vi "Scanner-Indentify-All-Action_Api.vi"(4 "加速度 (回頭)":dbl=700.0 format="%#_13g", 6 "最高速 (回頭)":dbl=800.0 format="%#_13g", 7 "Barcode數量":i32, 8 "Error In":errorcluster, 9 "加速度":dbl=700.0 format="%#_13g", 11 "最高速":dbl=800.0 format="%#_13g") -> (0 "error out":errorcluster, 1 "辨識機率":dbl[](array[slide]) scale=0.0..5.0, 2 "辨識機率":T1, 3 "輸出顏色-位置":T2(array[cluster]), 5 "總辨識結果":string[](array[string]))   [LabVIEW 2019]
uses:
  <vilib>/myRIO/Instrument Drivers/Onboard IO/DIO/typedefs/DIO Reference.ctl
  <vilib>/myRIO/Common/Instrument Driver Framework/Utilities/typedefs/myRIO Generic Hardware Reference.ctl
  <vilib>/myRIO/Common/Instrument Driver Framework/Utilities/typedefs/Hardware Version Enum.ctl
  <vilib>/myRIO/Common/Instrument Driver Framework/Utilities/typedefs/myRIO v1.0 Reference.ctl
  <vilib>/myRIO/Common/Instrument Driver Framework/Utilities/typedefs/Generic FPGA Reference.ctl
  <vilib>/myRIO/Common/Instrument Driver Framework/myRIO v1.0/DIO/typedefs/DIO Channels List.ctl
  <vilib>/myRIO/Common/Instrument Driver Framework/myRIO v1.0/DIO/typedefs/DIO Channels Enum.ctl
  <vilib>/userDefined/High Color/nirio_resource_hc.ctl
  <vilib>/myRIO/Common/Instrument Driver Framework/Utilities/vis/Is FPGA Ref Available.vi
  <vilib>/myRIO/Common/Instrument Driver Framework/myRIO v1.0/DIO/vis/myRIO v1.1 Open DIO.vi
  <vilib>/myRIO/Instrument Drivers/Onboard IO/DIO/vis/Write.vi
  b00342f0-89ff-48b8-870a-2e0bf58d2d45.vi
  <vilib>/myRIO/Common/Instrument Driver Framework/Utilities/vis/Validate Channels.vi
  <vilib>/myRIO/Common/Instrument Driver Framework/myRIO v1.0/DIO/vis/myRIO v1.0 Reserve DIO.vi
  <vilib>/myRIO/Common/Instrument Driver Framework/myRIO v1.0/Resource Manager/vis/myRIO v1.0 Reserve Channel List.vi
  <vilib>/myRIO/Common/Instrument Driver Framework/myRIO v1.0/DIO/vis/myRIO v1.0 Build MUX Configuration DIO.vi
  <vilib>/myRIO/Common/Instrument Driver Framework/myRIO v1.0/Resource Manager/vis/myRIO v1.0 Reserve Channel.vi
  <vilib>/myRIO/Common/Instrument Driver Framework/myRIO v1.0/Resource Manager/vis/myRIO v1.0 Unreserve Channel.vi
  <vilib>/myRIO/Common/Instrument Driver Framework/myRIO v1.0/Resource Manager/vis/myRIO v1.0 Create Configuration List.vi
  <vilib>/myRIO/Common/Instrument Driver Framework/myRIO v1.0/Resource Manager/vis/myRIO v1.0 Build Mutex Name.vi
  <vilib>/Utility/VariantDataType/GetNumericInfo.vi
  <vilib>/Utility/error.llb/Error Cluster From Error Code.vi
  <vilib>/myRIO/Common/Instrument Driver Framework/myRIO v1.0/myRIO v1.1 Open.vi
  <vilib>/myRIO/Common/Instrument Driver Framework/Utilities/vis/IO Manager.vi
  <vilib>/myRIO/Common/Instrument Driver Framework/Utilities/vis/Configuration Manager.vi
  <vilib>/myRIO/Common/Instrument Driver Framework/myRIO v1.0/Resource Manager/vis/myRIO v1.0 Configure IO.vi
  <vilib>/myRIO/Common/Instrument Driver Framework/myRIO v1.0/myRIO v1.0 Close.vi
  <vilib>/myRIO/Common/Instrument Driver Framework/myRIO v1.0/DIO/vis/myRIO v1.0 Write DIO.vi
  <vilib>/myRIO/Express VI/Onboard Devices/LED/LED Express VI.xnode
  <vilib>/myRIO/Instrument Drivers/Onboard IO/DIO/vis/myRIO DIO Open.xnode
  <vilib>/myRIO/Instrument Drivers/Onboard IO/DIO/DIO.lvlib
panel:
  in  "Tab Control":enum32{"Page 1", "Page 2", "Page 3"}(tab)
  out "第一次辨識機率":i32[](graph)
  out "第二次辨識結果":i32[](graph)
  out "總辨識機率 2":i32[](graph)
  out "總辨識機率":i32[](array[numeric])
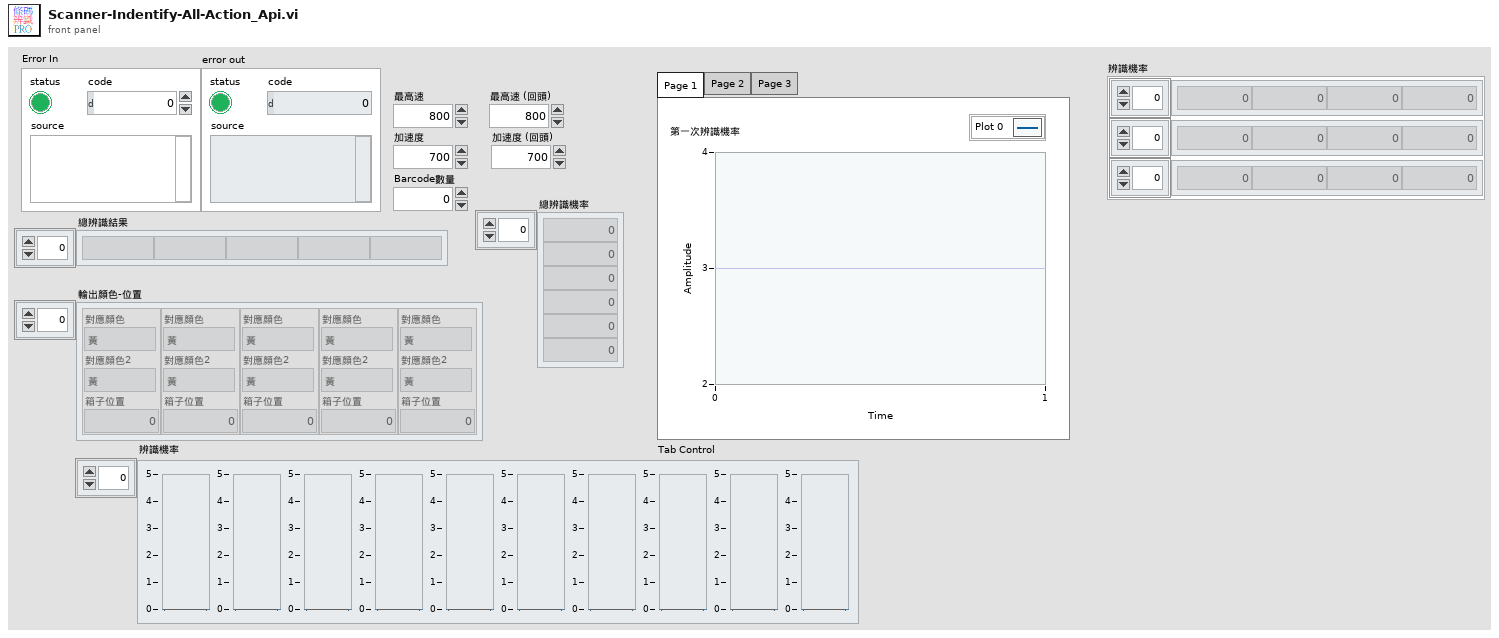
[diagram p1: front panel]
types:
  T1 = cluster{"Array":i32[], "Array":i32[], "Array":i32[]}
  T2 = cluster{"對應顏色":enum16{"黃", "紅", "綠", "藍", "黑", "無"}, "對應顏色2":enum16{"黃", "紅", "綠", "藍", "黑", "無"}, "箱子位置":i32}[]
  T3 = enum16{"前", "後", "オ", "右", "無", "0", "1", "2", "3", "4", "5", "6", "7"}
  T4 = typedef "DIO.lvlib/DIO Reference.ctl" = cluster{"myRIO Reference":T5, "DIO Channels List":T9}
  T5 = typedef "myRIO Generic Hardware Reference.ctl" = cluster{"myRIO Model":T6, "myRIO Hardware Reference":T7}
  T6 = typedef "Hardware Version Enum.ctl" = enum16{"Unknown", "myRIO-1900", "myRIO-1950", "roboRIO", "NI ELVIS RIO CM", "ELVIS III"}
  T7 = typedef "myRIO v1.0 Reference.ctl" = cluster{"Generic FPGA Reference":T8, "Allow multiple opens":bool}
  T8 = typedef "Generic FPGA Reference.ctl" = refnum<k20>
  T9 = typedef "DIO Channels List.ctl" = T10[]
  T10 = typedef "DIO Channels Enum.ctl" = enum16{"Not Connected", "C/DIO0", "C/DIO1", "C/DIO2", "C/DIO3", "C/DIO4", "C/DIO5", "C/DIO6", "C/DIO7", "A/DIO0", "A/DIO1", "A/DIO2", "A/DIO3", "A/DIO4", "A/DIO5", "A/DIO6", "A/DIO7", "A/DIO8", "A/DIO9", "A/DIO10", "A/DIO11", "A/DIO12", "A/DIO13", "A/DIO14", "A/DIO15", "A/DIO16", "A/DIO17", "A/DIO18", "A/DIO19", "B/DIO0", "B/DIO1", "B/DIO2", "B/DIO3", "B/DIO4", "B/DIO5", "B/DIO6", "B/DIO7", "B/DIO8", "B/DIO9", "B/DIO10", "B/DIO11", "B/DIO12", "B/DIO13", "B/DIO14", "B/DIO15", "B/DIO16", "B/DIO17", "B/DIO18", "B/DIO19", "LED0", "LED1", "LED2", "LED3", "Button0", "DIO/DIO0", "DIO/DIO1", "DIO/DIO2", "DIO/DIO3", "DIO/DIO4", "DIO/DIO5", "DIO/DIO6", "DIO/DIO7", "DIO/DIO8", "DIO/DIO9", "SPI/CS0", "SPI/CS1", "SPI/CS2", "SPI/CS3", "LED RADIO (Green)", "LED RADIO (Red)", "LED COMM (Green)", "LED COMM (Red)", "LED MODE (Green)", "LED MODE (Red)"}
  T11 = typedef "nirio_resource_hc.ctl" = tag
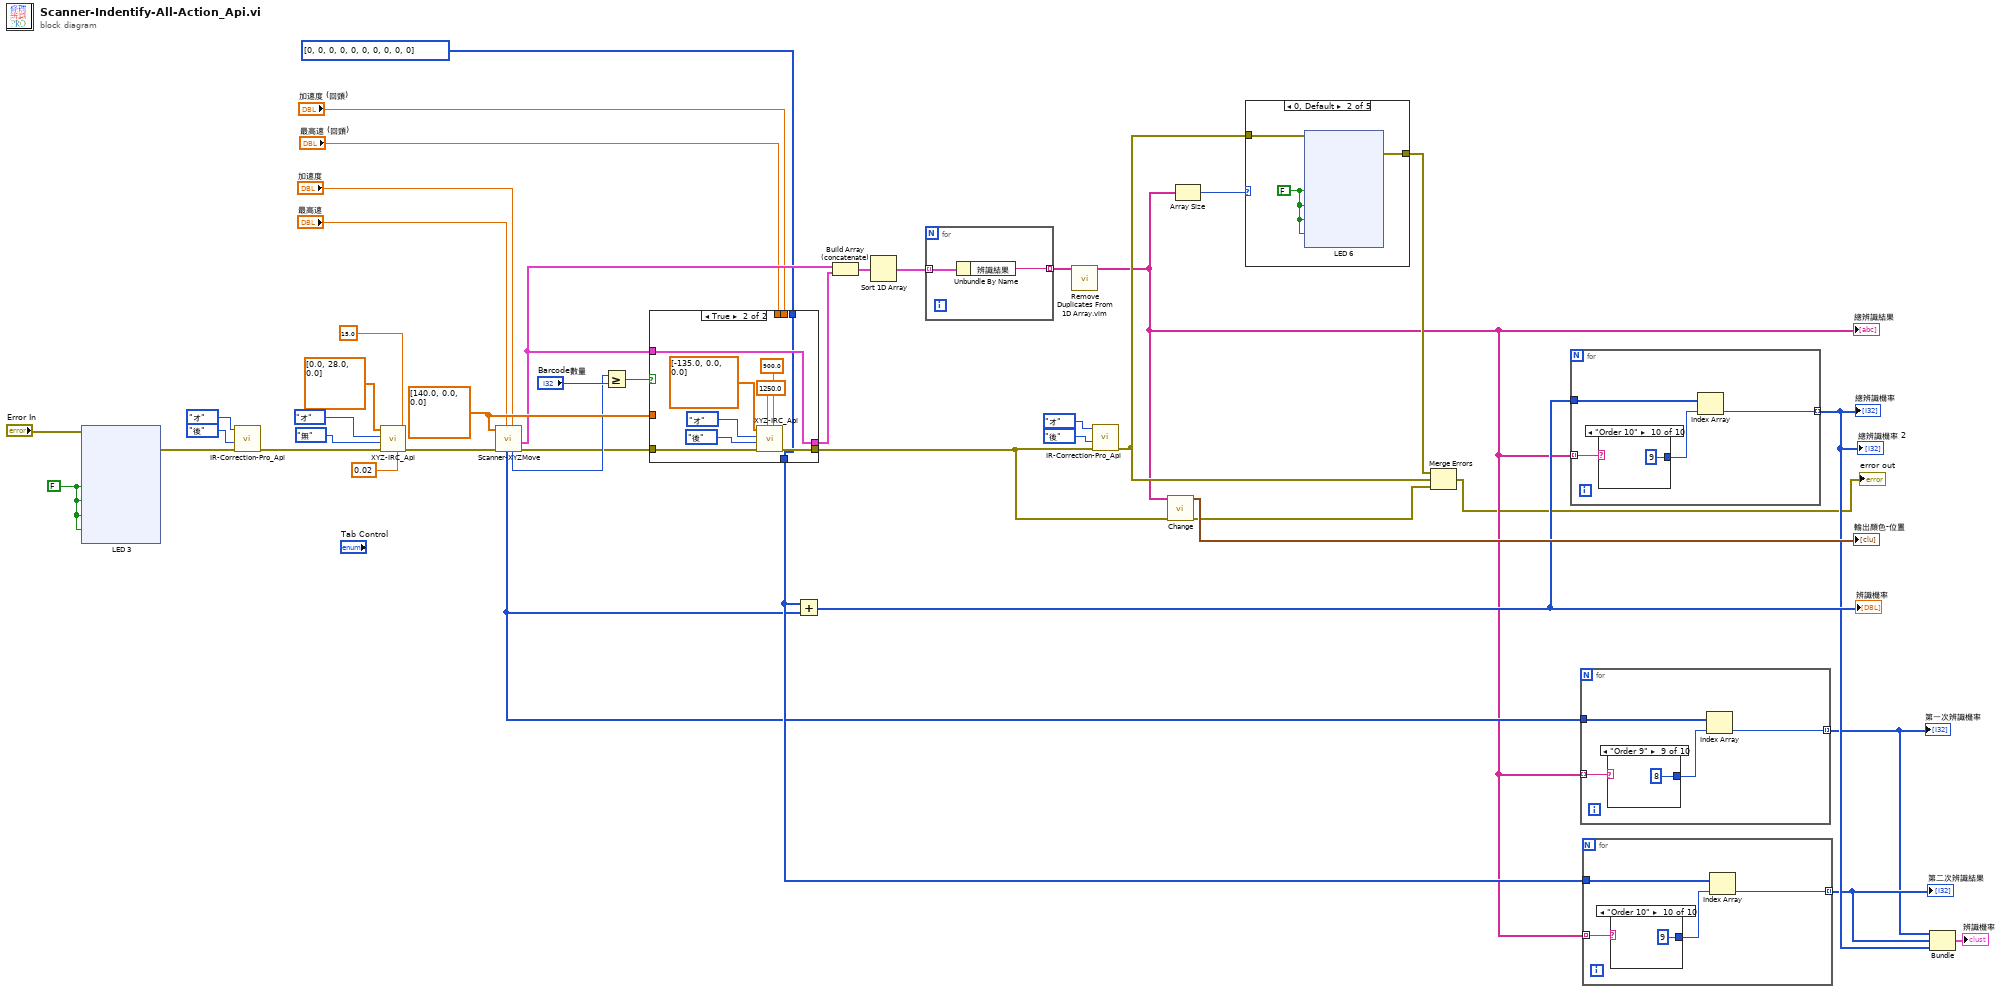
[diagram p0: block diagram]
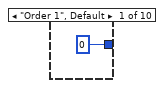
[diagram p2: hidden frame]
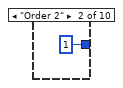
[diagram p3: hidden frame]
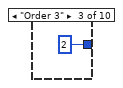
[diagram p4: hidden frame]
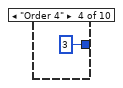
[diagram p5: hidden frame]
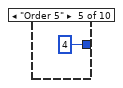
[diagram p6: hidden frame]
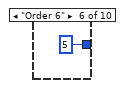
[diagram p7: hidden frame]
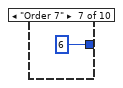
[diagram p8: hidden frame]
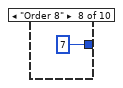
[diagram p9: hidden frame]
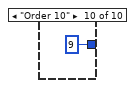
[diagram p10: hidden frame]
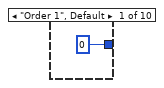
[diagram p11: hidden frame]
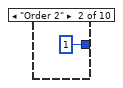
[diagram p12: hidden frame]
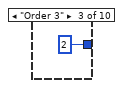
[diagram p13: hidden frame]
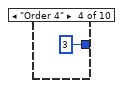
[diagram p14: hidden frame]
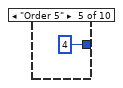
[diagram p15: hidden frame]
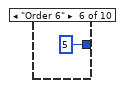
[diagram p16: hidden frame]
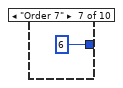
[diagram p17: hidden frame]
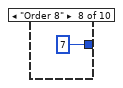
[diagram p18: hidden frame]
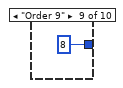
[diagram p19: hidden frame]
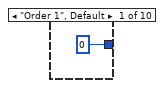
[diagram p20: hidden frame]
diagram:
  w21 = FALSE ("LED3")
  w42 = dbl[] [140.0, 0.0, 0.0] ("X-Y-Z移動")
  n1 = xnode "LED 3"("LED0"=w21, "LED1"=w21, "LED2"=w21, "LED3"=w21, "error in (no error)"="Error In") -> ("error out"=w19:errorcluster)
  n2 = call "IR-Correction-Pro_Api.vi"("Error In"=w19, "副邊校正"=T3."後", "主編校正"=enum16{"前", "後", "オ", "右", "無"}."オ") -> ("Error Out"=w32:errorcluster)  [unwired: 8 in]
  n3 = call "XYZ-IRC_Api.vi"("精準度"=15.0, "ExitRange"=0.02, "Error"=w32, "副邊校正"=T3."無", "主編校正"=enum16{"前", "後", "オ", "右", "無"}."オ", "X-Y-Z移動"=dbl[] [0.0, 28.0, 0.0]) -> ("Error Out"=w29:errorcluster)  [unwired: 5 in]
  n4 = call "Scanner-XYZMove.vi"("加速度"="加速度", "最高速"="最高速", "Error In"=w29, "X-Y-Z移動"=w42) -> ("Error Out"=w9:errorcluster, "辨識結果(包含位置)"=w18:cluster{"讀取到時的位子":dbl, "辨識結果":string}[], "辨識數量"=w15:i32, "讀取機率"=w4:i32[])  [unwired: 2 in, 2 out]
  n5 = Greater Or Equal?(x=w15, y="Barcode數量") -> (x >= y?=w16:bool)
  n6 = case shown="True" w16 {
    tunnel: w42 -> [w51 _]
    tunnel: [w50 w59] -> w40
    tunnel: [w49 w60] -> w37
    tunnel: w9 -> [w48 w61]
    tunnel: w18 -> [_ w59]
    tunnel: "加速度 (回頭)" -> [w47 _]
    tunnel: "最高速 (回頭)" -> [w46 _]
    tunnel: [w45 w53] -> w8
    tunnel: i32[] [0, 0, 0, 0, 0, 0, 0, 0, 0, 0] -> [_ w53]
    frame False {
      n7 = call "Scanner-XYZ-Back.vi"("加速度"=w47, "最高速"=w46, "Error In"=w48, "第一次位移"=w51, "X-Y-Z移動"=dbl[] [-140.0, 0.0, 0.0]) -> ("Error Out"=w49:errorcluster, "辨識結果(包含位置)"=w50:cluster{"讀取到時的位子":dbl, "辨識結果":string}[], "辨識機率"=w45:i32[])  [unwired: 2 in, 2 out]
    }
    frame True {
      n8 = call "XYZ-IRC_Api.vi"("加速度"=900.0, "最高速"=1250.0, "Error"=w61, "副邊校正"=T3."後", "主編校正"=enum16{"前", "後", "オ", "右", "無"}."オ", "X-Y-Z移動"=dbl[] [-135.0, 0.0, 0.0]) -> ("Error Out"=w60:errorcluster)  [unwired: 5 in]
    }
  }
  n9 = Add(x=w8, y=w4) -> (x+y=w10:i32[])
  "辨識機率" <- w10
  n10 = Build Array (concatenate)(w18, w40) -> (w41:cluster{"讀取到時的位子":dbl, "辨識結果":string}[])
  n11 = Sort 1D Array(array=w41) -> (sorted array=w39:cluster{"讀取到時的位子":dbl, "辨識結果":string}[])
  n12 = for {
    tunnel: w39 -> [w63] mode=indexing
    tunnel: [w62] -> w38 mode=indexing
    n13 = Unbundle By Name(w63) -> ("辨識結果"=w62:string)
  }
  n14 = call "Remove Duplicates From 1D Array.vim"("array"=w38) -> ("array with duplicates removed"=w2:string[])  [unwired: 10 in]
  "總辨識結果" <- w2
  n15 = call "IR-Correction-Pro_Api.vi"("Error In"=w37, "副邊校正"=T3."後", "主編校正"=enum16{"前", "後", "オ", "右", "無"}."オ") -> ("Error Out"=w28:errorcluster)  [unwired: 8 in]
  n16 = call "Change.vi"("Error In"=w37, "總辨識結果"=w2) -> ("Error Out"=w35:errorcluster, "輸出顏色-位置"=→"輸出顏色-位置":T2)  [unwired: 8 in]
  n17 = Array Size(array=w2) -> (size(s)=w31:i32)
  n18 = case shown="0, Default" w31 {
    tunnel: w28 -> [w66 w107 w147 w185 w225]
    tunnel: [w65 w106 w146 w184 w224] -> w30
    frame 4 {
      w64 = TRUE ("LED3")
      n19 = xnode "LED"("LED0"=w64, "LED1"=w64, "LED2"=w64, "LED3"=w64, "error in (no error)"=w66) -> ("error out"=w65:errorcluster)
    }
    frame 0, Default {
      w105 = FALSE ("LED2")
      n20 = xnode "LED 6"("LED0"=w105, "LED1"=w105, "LED2"=w105, "LED3"=w105, "error in (no error)"=w107) -> ("error out"=w106:errorcluster)
    }
    frame 1 {
      n21 = xnode "LED 5"("LED0"=TRUE ("LED2"), "error in (no error)"=w147) -> ("error out"=w146:errorcluster)
    }
    frame 2 {
      w186 = TRUE ("LED2")
      n22 = xnode "LED 4"("LED0"=w186, "LED1"=w186, "error in (no error)"=w185) -> ("error out"=w184:errorcluster)
    }
    frame 3 {
      w223 = TRUE ("LED2")
      n23 = xnode "LED 2"("LED0"=w223, "LED1"=w223, "LED2"=w223, "error in (no error)"=w225) -> ("error out"=w224:errorcluster)
    }
  }
  n24 = Merge Errors(w30, w28, w35) -> (→"error out":errorcluster)
  n25 = for {
    tunnel: w2 -> [w266] mode=indexing
    tunnel: w10 -> [w265]
    tunnel: [w263] -> w7 mode=indexing
    n26 = case shown="\"Order 10\"" w266 {
      tunnel: [0 1 2 3 4 5 6 7 8 9] -> w264
      frame "Order 1", Default {
      }
      frame "Order 2" {
      }
      frame "Order 3" {
      }
      frame "Order 4" {
      }
      frame "Order 5" {
      }
      frame "Order 6" {
      }
      frame "Order 7" {
      }
      frame "Order 8" {
      }
      frame "Order 9" {
      }
      frame "Order 10" {
      }
    }
    n27 = Index Array(array=w265, index=w264) -> (element=w263:i32)
  }
  "總辨識機率" <- w7
  "總辨識機率 2" <- w7
  n28 = for {
    tunnel: w4 -> [w280]
    tunnel: [w278] -> w3 mode=indexing
    tunnel: w2 -> [w277] mode=indexing
    n29 = case shown="\"Order 9\"" w277 {
      tunnel: [0 1 2 3 4 5 6 7 8 9] -> w279
      frame "Order 1", Default {
      }
      frame "Order 2" {
      }
      frame "Order 3" {
      }
      frame "Order 4" {
      }
      frame "Order 5" {
      }
      frame "Order 6" {
      }
      frame "Order 7" {
      }
      frame "Order 8" {
      }
      frame "Order 9" {
      }
      frame "Order 10" {
      }
    }
    n30 = Index Array(array=w280, index=w279) -> (element=w278:i32)
  }
  "第一次辨識機率" <- w3
  n31 = for {
    tunnel: w8 -> [w294]
    tunnel: [w292] -> w6 mode=indexing
    tunnel: w2 -> [w291] mode=indexing
    n32 = case shown="\"Order 10\"" w291 {
      tunnel: [0 1 2 3 4 5 6 7 8 9] -> w293
      frame "Order 1", Default {
      }
      frame "Order 2" {
      }
      frame "Order 3" {
      }
      frame "Order 4" {
      }
      frame "Order 5" {
      }
      frame "Order 6" {
      }
      frame "Order 7" {
      }
      frame "Order 8" {
      }
      frame "Order 9" {
      }
      frame "Order 10" {
      }
    }
    n33 = Index Array(array=w294, index=w293) -> (element=w292:i32)
  }
  "第二次辨識結果" <- w6
  n34 = Bundle(w3, w6, w7) -> (→"辨識機率":cluster{i32[], i32[], i32[]})  [unwired: 1 in]
